vi "Remover Peça.vi"(1 "Array Cluster in":T1(array[cluster])) -> (0 "Array Cluster out":T1(array[cluster]))   [LabVIEW 2020]
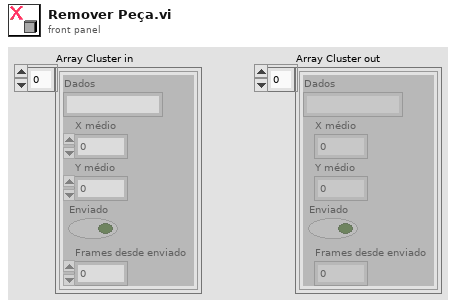
[diagram p1: front panel]
types:
  T1 = cluster{"Dados":string, "X médio":dbl, "Y médio":dbl, "Enviado":bool, "Frames desde enviado":dbl}[]
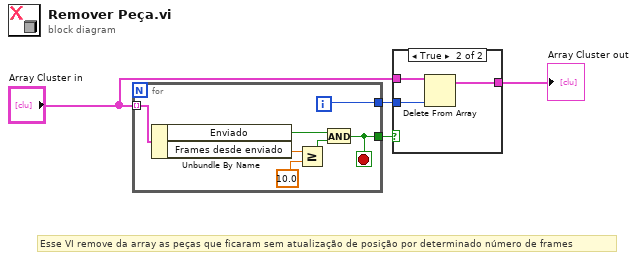
[diagram p0: block diagram]
diagram:
  # "Esse VI remove da array as peças que ficaram sem atualização de posição por determinado número de frames"
  n1 = for {
    tunnel: "Array Cluster in" -> [w9] mode=indexing
    tunnel: [w5] -> w1
    tunnel: [w8] -> w4
    i -> [w8]
    stop <- w5 stop-if-true
    n2 = Unbundle By Name(w9) -> ("Enviado"=w7:bool, "Frames desde enviado"=w11:dbl)
    n3 = Greater Or Equal?(x=w11, y=10.0) -> (x >= y?=w6:bool)
    n4 = And(x=w7, y=w6) -> (x .and. y?=w5:bool)
  }
  n5 = case shown="True" w1 {
    tunnel: "Array Cluster in" -> [w12 w15]
    tunnel: [w12 w14] -> w3
    tunnel: w4 -> [_ w13]
    frame False {
    }
    frame True {
      n6 = Delete From Array(array=w15, index=w13) -> (array with subset deleted=w14:T1)  [unwired: 1 in, 1 out]
    }
  }
  "Array Cluster out" <- w3
